vi "Enqueue Critical.vi"(8 "error in (no error)":errorcluster, 10 "Message":refnum<class "Message.lvclass">, 11 "Message Enqueuer in":refnum<class "Message Enqueuer.lvclass">) -> (0 "error out":errorcluster, 3 "Message Enqueuer out":refnum<class "Message Enqueuer.lvclass">)   [LabVIEW 2020, in "Actor Framework.lvlib" / "Message Enqueuer.lvclass"]
uses:
  Message Enqueuer.lvclass
  Message/Message.lvclass
  Message Enqueuer.lvclass/Message Enqueuer.ctl
  Message Priority Queue/Message Priority Queue.lvclass
  Message Priority.ctl
  Actor Framework.lvlib
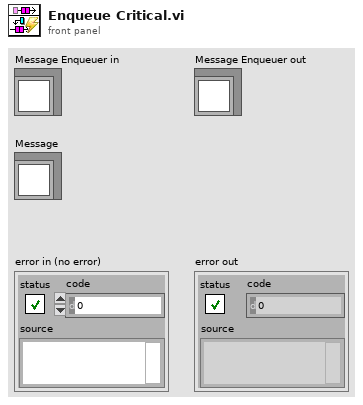
[diagram p1: front panel]
types:
  T1 = typedef "Actor Framework.lvlib/Message Enqueuer.lvclass/Message Priority.ctl" = enum16{"Low", "Normal", "High"}
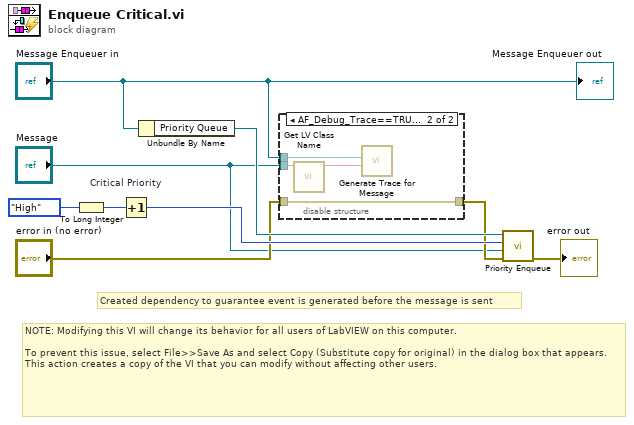
[diagram p0: block diagram]
diagram:
  # "Created dependency to guarantee event is generated before the message is sent"
  # "NOTE: Modifying this VI will change its behavior for all users of LabVIEW on this computer.\n\nTo prevent this issue, select File>>Save As and select Copy (Substitute copy for original) in the dialog box that appears. This action creates a copy of the VI that you can modify without affecting other users."
  n1 = To Long Integer(number=Message_Priority."High" ("Message Priority")) -> (32bit integer=w6:i32)
  n2 = Increment "Critical Priority"(x=w6) -> (x+1=w5:i32)
  n3 = Unbundle By Name("Message Enqueuer in") -> ("Priority Queue"=w9:refnum<class "Message Priority Queue.lvclass">)
  n4 = disable-structure shown="AF_Debug_Trace==TRUE" {
    disable-tunnel: "error in (no error)" -> [w10 w14]
    disable-tunnel: [w10 w14] -> w3
    disable-tunnel: "Message" -> [_ w13]
    disable-tunnel: "Message Enqueuer in" -> [_ w11]
    frame condition #0 (active) {
    }
    frame condition #1 {
      n5 = call <vilib>:"Get LV Class Name.vi"("object"=w13) -> ("class name"=w12:string)  [unwired: 9 in, 1 out]
      n6 = call "Generate Trace for Message.vi"("Message Name"=w12, "Receiver Enqueuer"=w11) -> ()  [unwired: 10 in]
    }
  }
  n7 = call "Priority Enqueue.vi"("error in (no error)"=w3, "Message"="Message", "priority"=w5, "Priority Queue in"=w9) -> ("error out"=→"error out":errorcluster)  [unwired: 6 in, 1 out]
  "Message Enqueuer out" <- "Message Enqueuer in"
